vi "vision communication test vi.vi"() -> ()   [LabVIEW 2009]
panel:
  in  "y locations":i16[](array[numeric])
  in  "x locations":i16[](array[numeric])
  out "x out":i16[](array[numeric])
  out "y out":i16[](array[numeric])
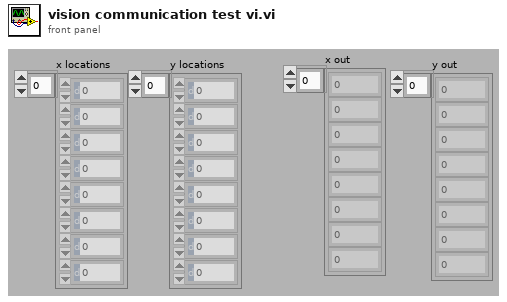
[diagram p1: front panel]
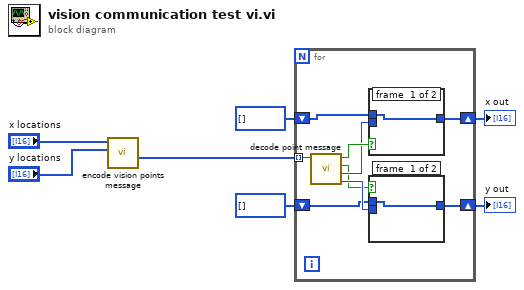
[diagram p0: block diagram]
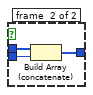
[diagram p2: hidden frame]
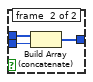
[diagram p3: hidden frame]
diagram:
  n1 = call "encode vision points message.vi"("y locations"="y locations", "x locations"="x locations") -> ("vision points message"=w1:u8[])  [unwired: 9 in]
  n2 = for {
    tunnel: w1 -> [w16] mode=indexing
    shift-right: [w13] -> w4
    shift-left: i16[] [] -> [w12]
    shift-right: [w9] -> w5
    shift-left: i16[] [] -> [w8]
    n3 = call "decode point message.vi"("input stream"=w16) -> ("y value"=w11:i16, "x value"=w14:i16, "new y"=w10:bool, "new x"=w15:bool)  [unwired: 6 in, 1 out]
    n4 = case shown="True" w15 {
      tunnel: w14 -> [_ w24]
      tunnel: [w21 w23] -> w13
      tunnel: w12 -> [w21 w22]
      frame #0 {
      }
      frame #1 {
        n5 = Build Array (concatenate)(w22, w24) -> (w23:i16[])
      }
    }
    n6 = case shown="True" w10 {
      tunnel: w11 -> [_ w20]
      tunnel: [w17 w19] -> w9
      tunnel: w8 -> [w17 w18]
      frame #0 {
      }
      frame #1 {
        n7 = Build Array (concatenate)(w18, w20) -> (w19:i16[])
      }
    }
  }
  "y out" <- w5
  "x out" <- w4
